vi "Check License.vi"() -> (1 "stripped path":path, 2 "s? t:f":string, 3 "校验成功":bool)   [LabVIEW 2013]
panel:
  in  "error in":errorcluster caption="错误输入（无错误）"
  out "error out":errorcluster caption="错误输出"
  out "MD5":string caption="License"
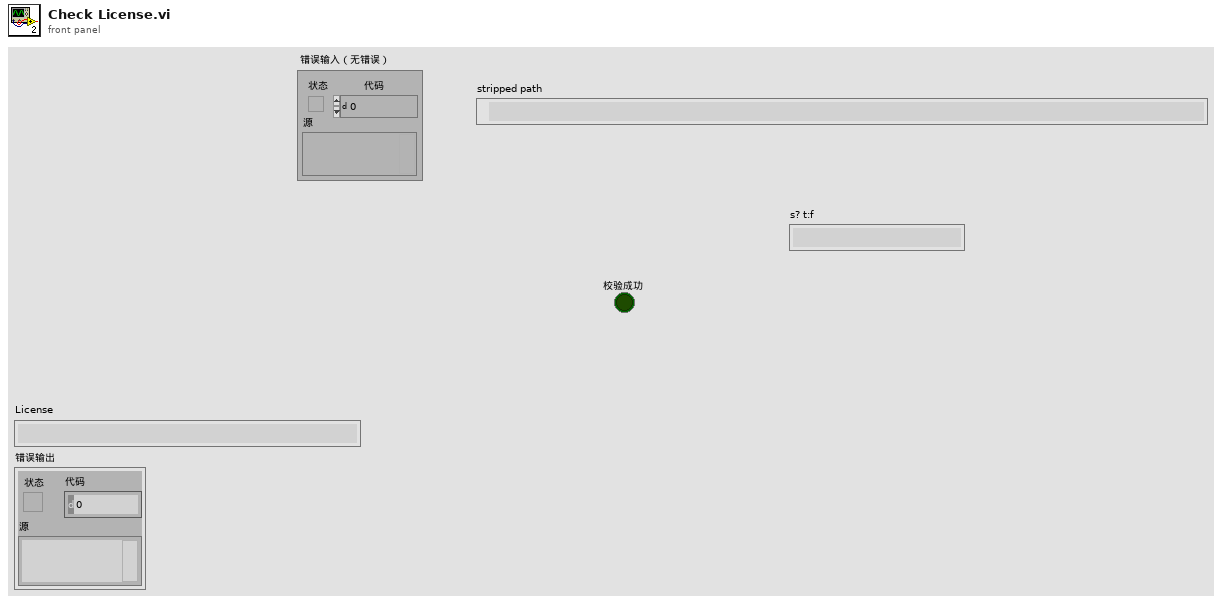
[diagram p1: front panel]
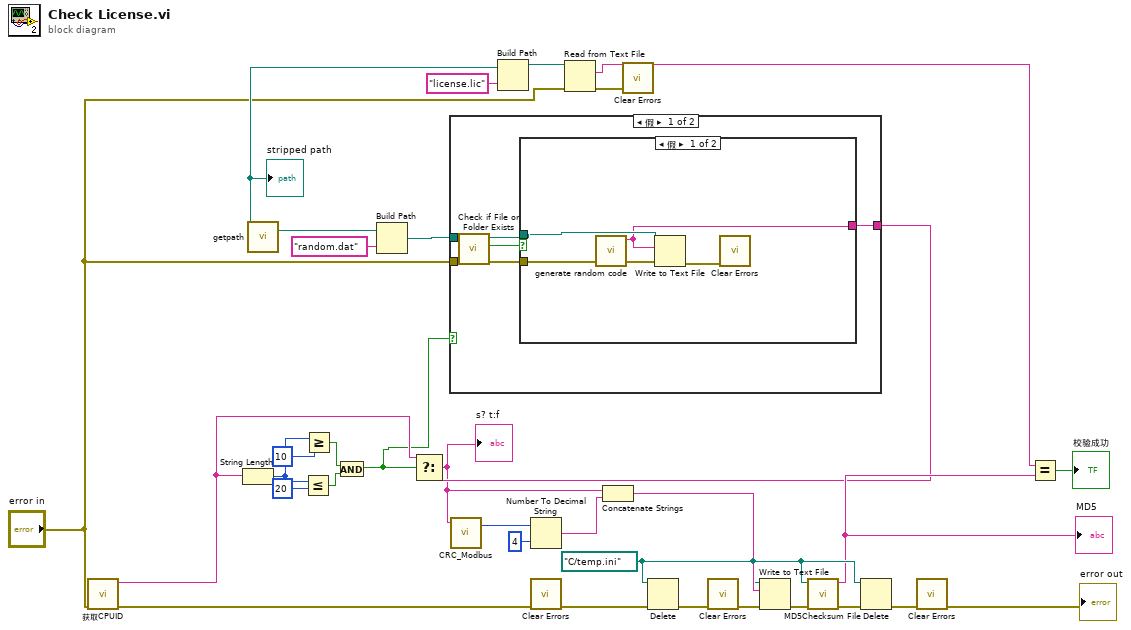
[diagram p0: block diagram]
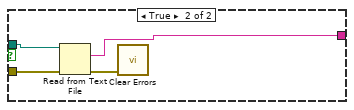
[diagram p2: hidden frame]
diagram:
  w26 = path "C:/temp.ini" ("文件（使用对话框）")
  n1 = call "获取CPUID.vi"("error in (no error)"="error in") -> ("error out"=w22:errorcluster, "CPU ID"=w2:string)  [unwired: 9 in]
  n2 = String Length(string=w2) -> (length=w8:i32)
  n3 = call "getpath.vi"() -> ("stripped path"=w13:path)  [unwired: 11 in]
  "stripped path" <- w13
  n4 = Less Or Equal?(x=w8, y=20) -> (x <= y?=w5:bool)
  n5 = Greater Or Equal?(x=w8, y=10) -> (x >= y?=w6:bool)
  n6 = And(x=w6, y=w5) -> (x .and. y?=w1:bool)
  n7 = Build Path(base path=w13, name or relative path="random.dat" ("名称或相对路径")) -> (appended path=w12:path)
  n8 = case shown="假" w1 {
    tunnel: w12 -> [w38 _]
    tunnel: "error in" -> [w34 _]
    tunnel: [w33 _] -> w4
    frame False {
      n9 = call <vilib>:"Check if File or Folder Exists.vi"("error in (no error)"=w34, "path"=w38) -> ("error out"=w35:errorcluster, "file or folder exists?"=w37:bool, "dup path"=w36:path)  [unwired: 7 in]
      n10 = case shown="假" w37 {
        tunnel: w36 -> [w42 w46]
        tunnel: w35 -> [w41 w45]
        tunnel: [w39 w43] -> w33
        frame False {
          n11 = call "generate random code.vi"() -> ("random code"=w39:string)  [unwired: 11 in]
          n12 = Write to Text File(file (use dialog)=w42, text=w39, error in=w41) -> (error out=w40:errorcluster)  [unwired: 1 in, 2 out]
          n13 = call <vilib>:"Clear Errors.vi"("error in (no error)"=w40) -> ()  [unwired: 6 in, 1 out]
        }
        frame True {
          n14 = Read from Text File(file (use dialog)=w46, error in=w45) -> (text=w43:string, error out=w44:errorcluster)  [unwired: 2 in, 2 out]
          n15 = call <vilib>:"Clear Errors.vi"("error in (no error)"=w44) -> ()  [unwired: 6 in, 1 out]
        }
      }
    }
    frame True {
    }
  }
  n16 = Select(t=w2, s=w1, f=w4) -> (s? t:f=w3:string)
  "s? t:f" <- w3
  n17 = call "CRC_Modbus.vi"("字符串"=w3) -> ("输出变量"=w32:u16)  [unwired: 10 in]
  n18 = Build Path(base path=w13, name or relative path="license.lic" ("名称或相对路径")) -> (appended path=w18:path)
  n19 = Number To Decimal String(number=w32, width (-)=i16 4 ("宽度(-)")) -> (decimal integer string=w30:string)
  n20 = call <vilib>:"Clear Errors.vi"("error in (no error)"=w22) -> ("error out"=w21:errorcluster)  [unwired: 6 in]
  n21 = Read from Text File(file (use dialog)=w18, error in="error in") -> (text=w17:string, error out=w10:errorcluster)  [unwired: 2 in, 2 out]
  n22 = Concatenate Strings(w3, w30) -> (w29:string)
  n23 = call <vilib>:"Clear Errors.vi"("error in (no error)"=w10) -> ()  [unwired: 6 in, 1 out]
  n24 = Delete(path (use dialog)=w26, error in=w21) -> (error out=w24:errorcluster)  [unwired: 3 in, 2 out]
  n25 = call <vilib>:"Clear Errors.vi"("error in (no error)"=w24) -> ("error out"=w23:errorcluster)  [unwired: 6 in]
  n26 = Write to Text File(file (use dialog)=w26, text=w29, error in=w23) -> (error out=w28:errorcluster)  [unwired: 1 in, 2 out]
  n27 = call <vilib>:"MD5Checksum File.vi"("error in (no error)"=w28, "Path"=w26) -> ("error out"=w27:errorcluster, "MD5 message-digest"=w16:string)  [unwired: 8 in]
  "MD5" <- w16
  n28 = Delete(path (use dialog)=w26, error in=w27) -> (error out=w25:errorcluster)  [unwired: 3 in, 2 out]
  n29 = call <vilib>:"Clear Errors.vi"("error in (no error)"=w25) -> ("error out"=→"error out":errorcluster)  [unwired: 6 in]
  n30 = Equal?(x=w17, y=w16) -> (x = y?=→"校验成功":bool)
